vi "Read Process Name Arr.vi"(8 "error in (no error)":errorcluster, 11 "Main Process Class in":refnum<class "Main Class.lvclass">) -> (0 "error out":errorcluster, 2 "Process Name Arr":variant, 3 "Main Process Class out":refnum<class "Main Class.lvclass">)   [LabVIEW 2019, in "Main Class.lvclass"]
uses:
  Main Class.lvclass
  Main Class.lvclass/Main Class.ctl
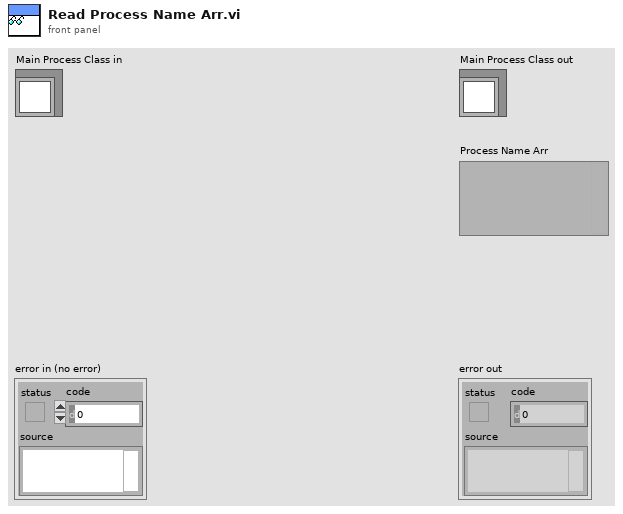
[diagram p1: front panel]
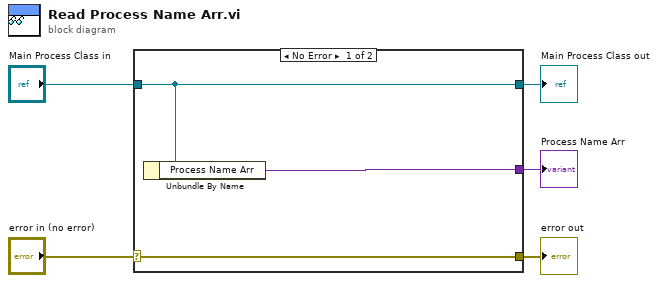
[diagram p0: block diagram]
diagram:
  n1 = case shown="No Error" "error in (no error)" {
    selector: "error in (no error)" -> [w8 w9]
    tunnel: [w8 w9] -> w4
    tunnel: [w7 w10] -> w2
    tunnel: "Main Process Class in" -> [w7 w10]
    tunnel: [w6 _] -> w1
    frame No Error {
      n2 = Unbundle By Name(w7) -> ("Process Name Arr"=w6:variant)
    }
    frame Error {
    }
  }
  "error out" <- w4
  "Main Process Class out" <- w2
  "Process Name Arr" <- w1
